vi "HelioNoise.vi"() -> ()   [LabVIEW 2010]
uses:
  bricks/classes/ImageCollection/ImageCollection.lvclass
  <vilib>/Analysis/NI_AALBase.lvlib
  bricks/classes/ImageCollection/add_mode_enum.ctl
  bricks/classes/Image/Image.lvclass
  bricks/classes/Image/storage_mode.ctl
  <vilib>/vision/Image Controls.llb/IMAQ Image.ctl
panel:
  in  "loadROIsButton":bool
  in  "saveROIsButton":bool
  out "DS/S vs. S (bg subtracted)":cluster{dbl, dbl}[](graph) caption="DS/S vs. S (background subtracted)"
  in  "saveButton":bool
  out "files to process":i32
  out "progress":u8(slide) scale=0.0..100.0
  in  "pattern":string="*channel01.tif"
  out "ROIs":T1(plugin-control)
  out "DS/S vs. S (bg NOT subtracted)":cluster{dbl, dbl}[](graph) caption="DS/S vs. S (background NOT subtracted from S)"
  in  "stopButton":bool
  in  "path":path
  in  "runButton":bool
  # "Noise Analyser"
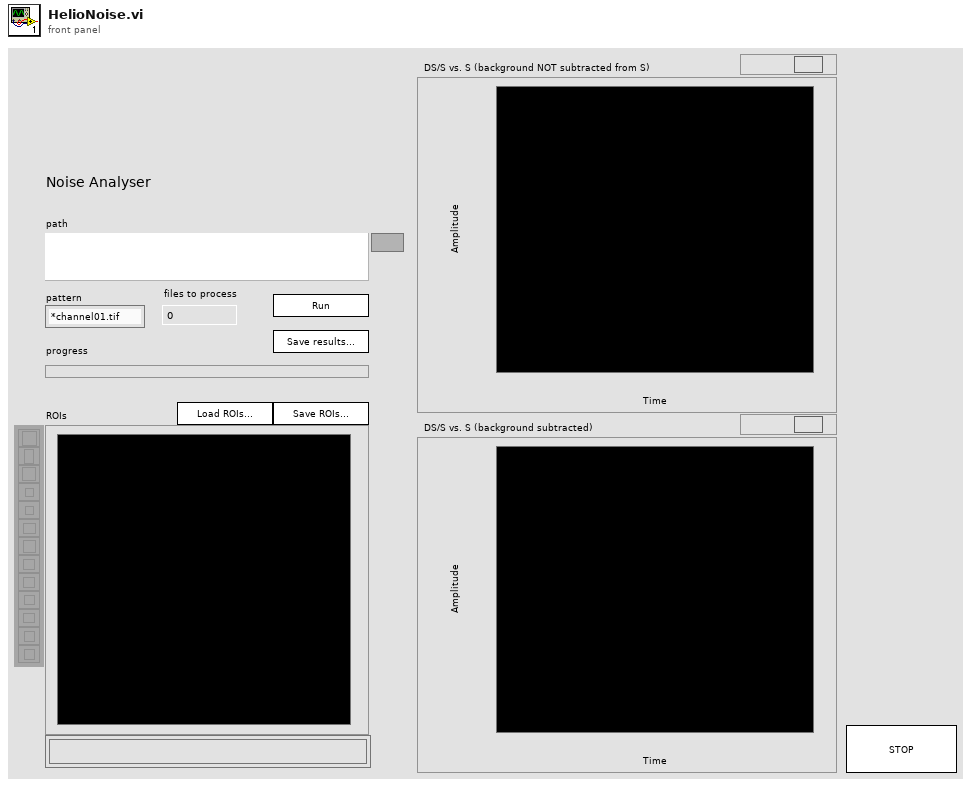
[diagram p1: front panel]
types:
  T1 = typedef "IMAQ Image.ctl" = refnum<image>
  T2 = typedef "Image.lvclass/storage_mode.ctl" = enum16{"RAM", "disk"}
  T3 = typedef "ImageCollection.lvclass/add_mode_enum.ctl" = enum16{"instance", "copy"}
  T4 = typedef "ROI Descriptor" = cluster{"Global Rectangle":i32[], "Contours":cluster{"ID":enum32{"External", "Internal"}, "Type":u32, "Coordinates":i32[]}[]}
  T5 = cluster{"Global Rectangle":i32[], "Contours":cluster{"Contour Type":u32, "ROI Type":u32, "Points":i32[]}[]}
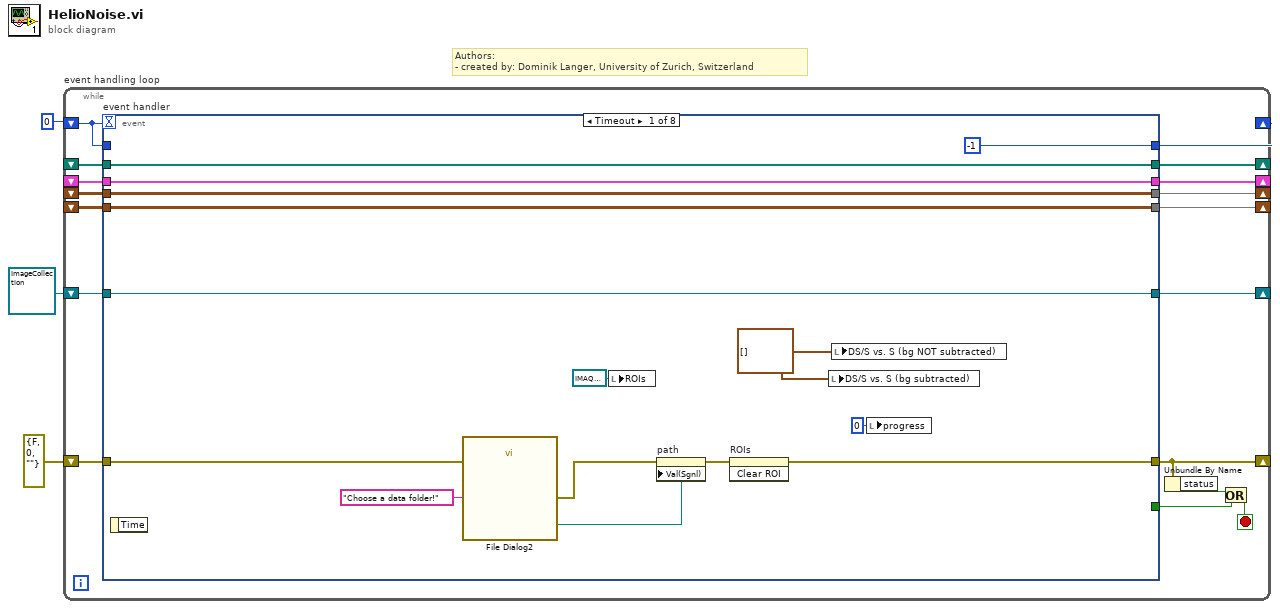
[diagram p0: block diagram]
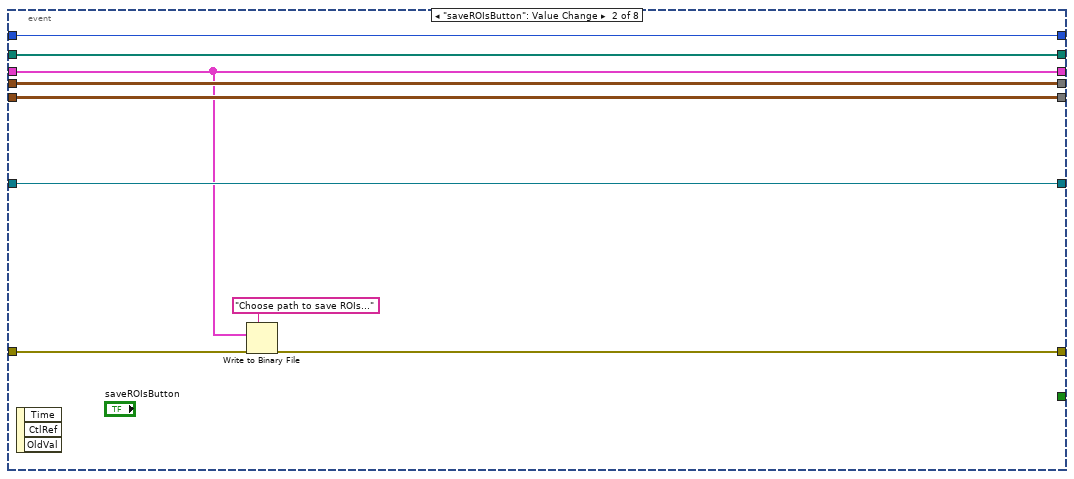
[diagram p2: hidden frame]
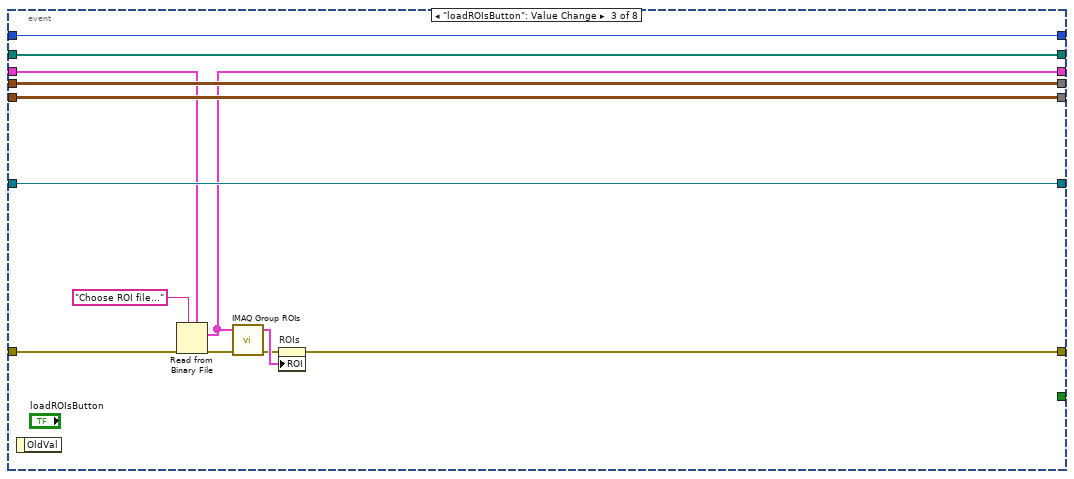
[diagram p3: hidden frame]
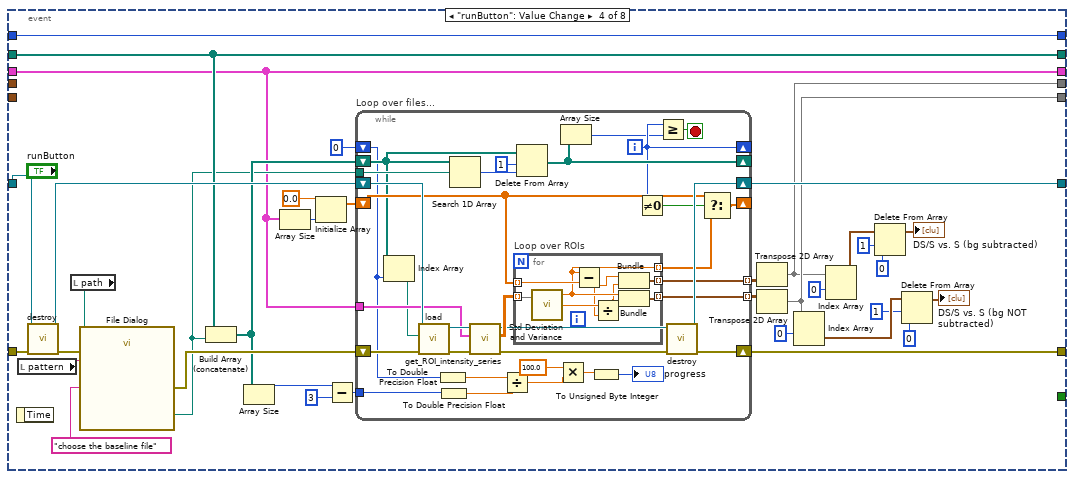
[diagram p4: hidden frame]
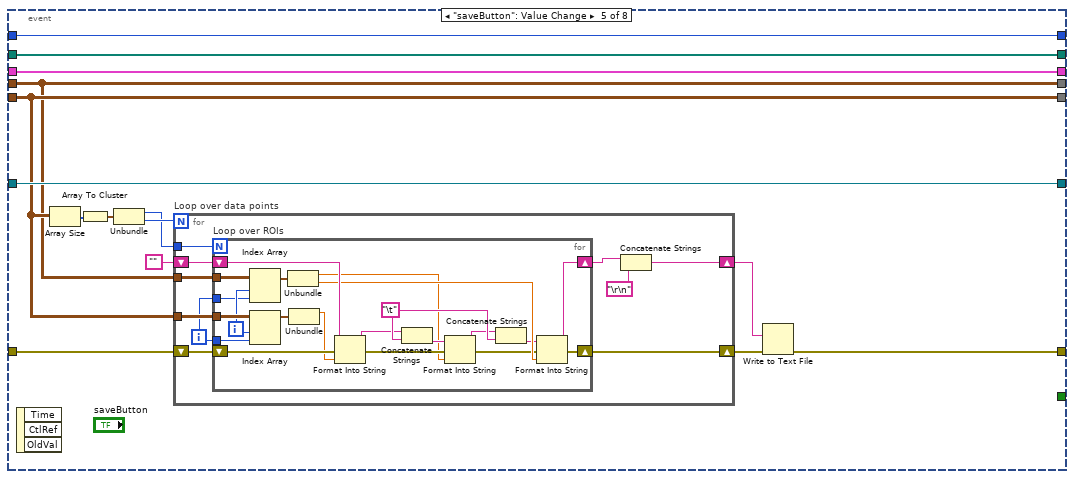
[diagram p5: hidden frame]
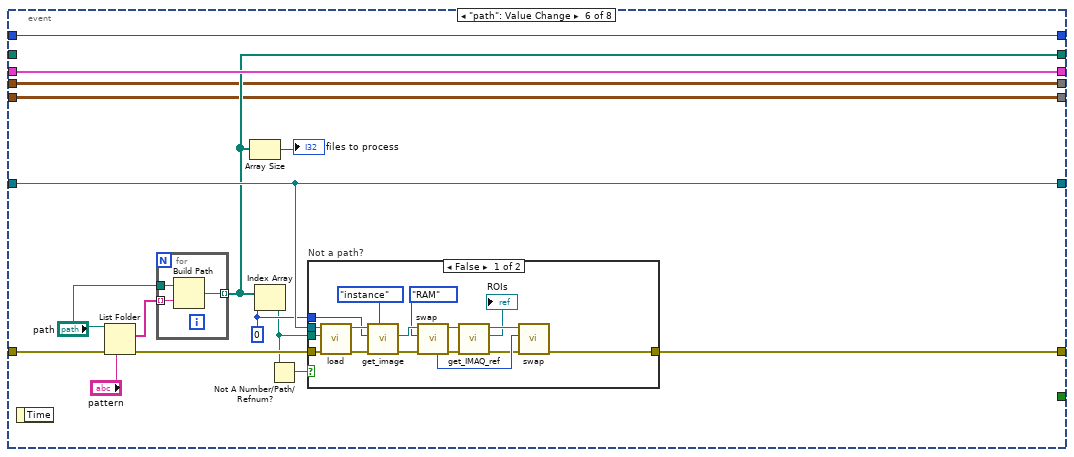
[diagram p6: hidden frame]
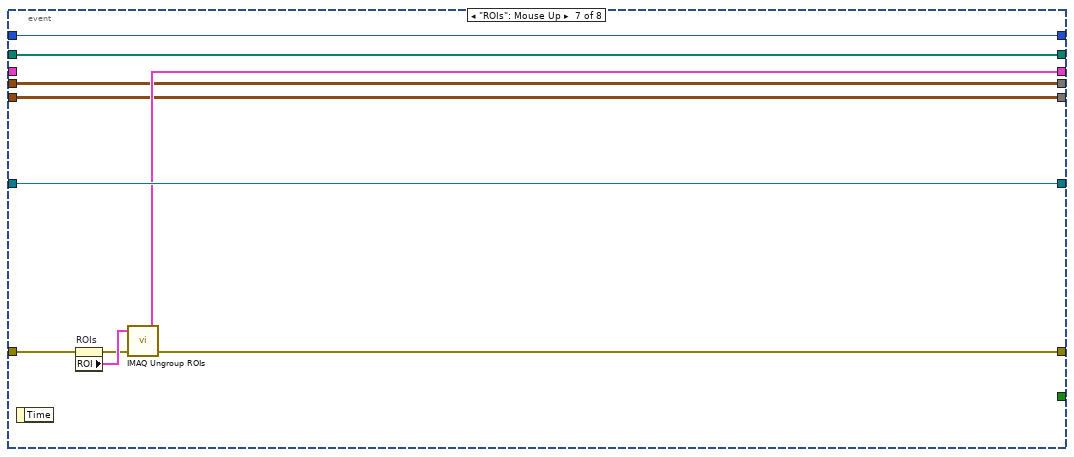
[diagram p8: hidden frame]
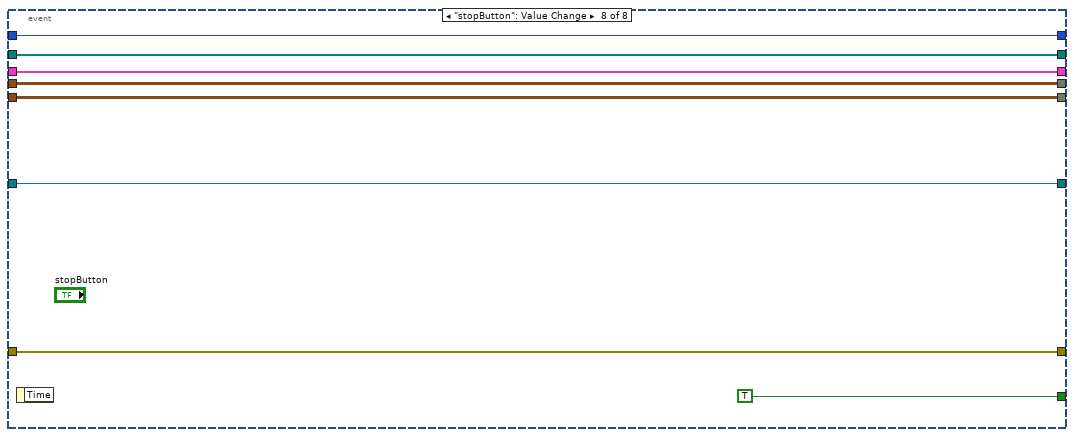
[diagram p9: hidden frame]
diagram:
  # "Authors: \n- created by: Dominik Langer, University of Zurich, Switzerland"
  n1 = while "event handling loop" {
    shift-right: [w15] -> _
    shift-left: errorcluster {"status"=FALSE, "code"=0, "source"=""} ("error out") -> [w19]
    shift-right: [w18] -> _
    shift-left: refnum<class "ImageCollection.lvclass"> refnum ("ImageCollection.lvclass") -> [w20]
    shift-right: [w16] -> _
    shift-left: _ -> [w17]
    shift-right: [w10] -> _
    shift-left: 0 -> [w11]
    shift-right: [w9] -> _
    shift-left: _ -> [w8]
    shift-right: [w6] -> _
    shift-left: _ -> [w7]
    shift-right: [w5] -> _
    shift-left: _ -> [w4]
    stop <- w12 stop-if-true
    n2 = event "event handler" shown="[0] Timeout" {
      selector: _ -> [_ _ _ _ _ _ _ _]
      dyn-events: _ -> [_ _ _ _ _ _ _ _]
      timeout: w11 -> [_ _ _ _ _ _ _ _]
      tunnel: w20 -> [w35 w44 w57 w89 w149 w192 w227 w234]
      tunnel: w19 -> [w27 w39 w52 w90 w144 w196 w226 w235]
      tunnel: [w22 w38 w49 w93 w142 w190 w223 w235] -> w15
      tunnel: [w35 w44 w57 w92 w149 w192 w227 w234] -> w18
      tunnel: [_ _ _ _ _ _ _ TRUE] -> w14
      tunnel: w17 -> [w34 w43 w56 w83 w148 _ w222 w232]
      tunnel: [w34 w43 w56 w83 w148 w184 w222 w232] -> w16
      tunnel: [-1 w42 w55 w91 w147 w186 w221 w231] -> w10
      tunnel: w11 -> [_ w42 w55 w91 w147 w186 w221 w231]
      tunnel: [w31 w37 w48 w72 w146 w185 w220 w230] -> w9
      tunnel: w8 -> [w31 w37 w51 w72 w146 w185 _ w230]
      tunnel: w7 -> [w29 w41 w54 _ w140 w182 w219 w229]
      tunnel: [w29 w41 w54 w68 w140 w182 w219 w229] -> w6
      tunnel: [w28 w40 w53 w60 w135 w181 w218 w228] -> w5
      tunnel: w4 -> [w28 w40 w53 _ w135 w181 w218 w228]
      event Timeout {
        w21 = cluster{dbl, dbl}[] [] ("XY Graph")
        n3 = event-data() -> ()  [unwired: 1 in, 1 out]
        n4 = call "File Dialog2"("prompt"="Choose a data folder!", "error in"=w27) -> ("selected path"=w25:path, "error out"=w26:errorcluster)  [unwired: 10 in, 2 out]
        n5 = local write "ROIs"(T1 refnum ("Image")) -> ()
        n6 = property on="path" class="Path"(error in=w26, "Val(Sgnl)"=w25) -> (error out=w23:errorcluster)  [unwired: 1 in, 1 out]
        n7 = invoke on="ROIs" class="ImageControl" method="Clear ROI"(error in=w23) -> (error out=w22:errorcluster)  [unwired: 2 in, 2 out]
        n8 = local write "DS/S vs. S (bg subtracted)"(w21) -> ()
        n9 = local write "DS/S vs. S (bg NOT subtracted)"(w21) -> ()
        n10 = local write "progress"(u8 0 ("progress")) -> ()
      }
      event "saveROIsButton": Value Change {
        n11 = event-data() -> ()  [unwired: 1 in, 3 out]
        n12 = Write to Binary File(data=w37, error in=w39, 7:"Choose path to save ROIs..." ("prompt (Choose or enter file path)")) -> (error out=w38:errorcluster)  [unwired: 3 in, 2 out]
      }
      event "loadROIsButton": Value Change {
        n13 = event-data() -> ()  [unwired: 1 in, 1 out]
        n14 = Read from Binary File(5:w51, 7:"Choose ROI file..." ("prompt (Open existing file)"), 8:w52) -> (0:w46:errorcluster, 2:w48:T4[])  [unwired: 3 in, 2 out]
        n15 = call "IMAQ Group ROIs"("error in (no error)"=w46, "ROI Descriptors"=w48) -> ("error out"=w45:errorcluster, "ROI Descriptor out"=w47:T4)  [unwired: 2 in]
        n16 = property on="ROIs" class="ImageControl"(error in=w45, "ROI"=w47) -> (error out=w49:errorcluster)  [unwired: 1 in, 1 out]
      }
      event "runButton": Value Change {
        n17 = event-data() -> ()  [unwired: 1 in, 1 out]
        n18 = local read "pattern"() -> (w77:string)
        n19 = call-dynamic "destroy.vi"("error in (no error)"=w90, "ImageCollection in"=w89) -> ("error out"=w85:errorcluster, "ImageCollection out"=w88:refnum<class "ImageCollection.lvclass">)  [unwired: 8 in]
        n20 = local read "path"() -> (w78:path)
        n21 = call "File Dialog"("start path"=w78, "prompt"="choose the baseline file", "error in"=w85, "pattern (all files)"=w77) -> ("selected path"=w75:path, "error out"=w84:errorcluster)  [unwired: 8 in, 2 out]
        n22 = Build Array (concatenate)(w83, w75) -> (w76:path[])
        n23 = Array Size(array=w76) -> (size(s)=w66:i32)
        n24 = Array Size(array=w72) -> (size(s)=w73:i32)
        n25 = Initialize Array(0.0 ("element"), w73) -> (w70:dbl[])
        n26 = Subtract(x=w66, y=3) -> (x-y=w65:i32)
        n27 = while "Loop over files..." {
          shift-right: [w120] -> w93
          shift-left: w84 -> [w125]
          tunnel: [w108] -> w87 mode=indexing
          shift-right: [w118] -> w92
          shift-left: w88 -> [w126]
          tunnel: w72 -> [w117]
          shift-right: [w109] -> _
          shift-left: w70 -> [w107]
          shift-right: [w99] -> _
          shift-left: w76 -> [w103]
          tunnel: w75 -> [w106]
          shift-right: [w98] -> _
          shift-left: 0 -> [w100]
          tunnel: w65 -> [w95]
          tunnel: [w94] -> w64 mode=indexing
          i -> [w98]
          stop <- w97 stop-if-true
          n28 = Index Array(array=w103, index=w100) -> (element=w102:path)
          n29 = call "load.vi"("error in (no error)"=w125, "Path"=w102, "ImageCollection in"=w126) -> ("error out"=w124:errorcluster, "ImageCollection out"=w123:refnum<class "ImageCollection.lvclass">)  [unwired: 5 in, 2 out]
          n30 = To Double Precision Float(number=w100) -> (double precision float=w116:dbl)
          n31 = To Double Precision Float(number=w95) -> (double precision float=w115:dbl)
          n32 = Search 1D Array(1D array=w103, element=w106) -> (index of element=w105:i32)  [unwired: 1 in]
          n33 = call "get_ROI_intensity_series.vi"("error in (no error)"=w124, "ROIs"=w117, "ImageCollection in"=w123) -> ("error out"=w121:errorcluster, "intensity series"=w122:dbl[][], "ImageCollection out"=w119:refnum<class "ImageCollection.lvclass">)  [unwired: 6 in]
          n34 = Divide(x=w116, y=w115) -> (x/y=w114:dbl)
          n35 = for "Loop over ROIs" {
            tunnel: w122 -> [w134] mode=indexing
            tunnel: [w131] -> w108 mode=indexing
            tunnel: [w130] -> w110 mode=indexing
            tunnel: w107 -> [w133] mode=indexing
            tunnel: [w129] -> w94 mode=indexing
            n36 = call <vilib>:"Std Deviation and Variance.vi"("X"=w134) -> ("mean"=w130:dbl, "standard deviation"=w132:dbl)  [unwired: 1 in, 1 out]
            n37 = Subtract(x=w130, y=w133) -> (x-y=w127:dbl)
            n38 = Divide(x=w132, y=w127) -> (x/y=w128:dbl)
            n39 = Bundle(w127, w128) -> (w129:cluster{dbl, dbl})  [unwired: 1 in]
            n40 = Bundle("mean"=w130, w128) -> (w131:cluster{"mean":dbl, dbl})  [unwired: 1 in]
          }
          n41 = Delete From Array(array=w103, length=1, index=w105) -> (array with subset deleted=w99:path[])  [unwired: 1 out]
          n42 = Multiply(x=100.0, y=w114) -> (x*y=w112:dbl)
          n43 = Array Size(array=w99) -> (size(s)=w96:i32)
          n44 = To Unsigned Byte Integer(number=w112) -> (unsigned 8bit integer=→"progress":u8)
          n45 = Not Equal To 0?(x=w98) -> (x != 0?=w101:bool)
          n46 = Greater Or Equal?(x=w98, y=w96) -> (x >= y?=w97:bool)
          n47 = call-dynamic "destroy.vi"("error in (no error)"=w121, "ImageCollection in"=w119) -> ("error out"=w120:errorcluster, "ImageCollection out"=w118:refnum<class "ImageCollection.lvclass">)  [unwired: 8 in]
          n48 = Select(t=w107, s=w101, f=w110) -> (s? t:f=w109:dbl[])
        }
        n49 = Transpose 2D Array(2D array=w64) -> (transposed array=w60:cluster{dbl, dbl}[][])
        n50 = Transpose 2D Array(2D array=w87) -> (transposed array=w68:cluster{"mean":dbl, dbl}[][])
        n51 = Index Array(array=w68, index (row)=0) -> (element=w82:cluster{"mean":dbl, dbl}[])  [unwired: 1 in]
        n52 = Index Array(array=w60, index (row)=0) -> (element=w58:cluster{dbl, dbl}[])  [unwired: 1 in]
        n53 = Delete From Array(array=w58, length=1, index=0) -> (array with subset deleted=→"DS/S vs. S (bg subtracted)":cluster{dbl, dbl}[])  [unwired: 1 out]
        n54 = Delete From Array(array=w82, length=1, index=0) -> (array with subset deleted=→"DS/S vs. S (bg NOT subtracted)":cluster{"mean":dbl, dbl}[])  [unwired: 1 out]
      }
      event "saveButton": Value Change {
        n55 = event-data() -> ()  [unwired: 1 in, 3 out]
        n56 = Array Size(array=w140) -> (size(s)=w139:i32[])
        n57 = Array To Cluster(array=w139) -> (cluster=w138:cluster{"[0]":i32, "[1]":i32})
        n58 = Unbundle(w138) -> ("[0]"=w136:i32, "[1]"=w137:i32)
        n59 = for "Loop over data points" {
          N: w137 -> [_]
          tunnel: w140 -> [w159]
          shift-right: [w153] -> w141
          shift-left: "" -> [w158]
          shift-right: [w156] -> w143
          shift-left: w144 -> [w157]
          tunnel: w136 -> [w155]
          tunnel: w135 -> [w151]
          i -> [w150]
          n60 = for "Loop over ROIs" {
            N: w155 -> [_]
            tunnel: w159 -> [w175]
            shift-right: [w176] -> w154
            shift-left: w158 -> [w177]
            shift-right: [w178] -> w156
            shift-left: w157 -> [w180]
            tunnel: w150 -> [w173]
            tunnel: w151 -> [w171]
            tunnel: w150 -> [w170]
            i -> [w172]
            w164 = "\t"
            n61 = Index Array(array=w171, index (row)=w172, index (col)=w170) -> (element=w169:cluster{dbl, dbl})
            n62 = Index Array(array=w175, index (row)=w172, index (col)=w173) -> (element=w174:cluster{"mean":dbl, dbl})
            n63 = Unbundle(w169) -> (w160:dbl, w168:dbl)
            n64 = Unbundle(w174) -> ("mean"=w179:dbl)  [unwired: 1 out]
            n65 = Format Into String(initial string=w177, error in=w180, w179) -> (resulting string=w162:string, error out=w167:errorcluster)  [unwired: 1 in]
            n66 = Concatenate Strings(w162, w164) -> (w165:string)
            n67 = Format Into String(initial string=w165, error in=w167, w160) -> (resulting string=w163:string, error out=w166:errorcluster)  [unwired: 1 in]
            n68 = Concatenate Strings(w163, w164) -> (w161:string)
            n69 = Format Into String(initial string=w161, error in=w166, w168) -> (resulting string=w176:string, error out=w178:errorcluster)  [unwired: 1 in]
          }
          n70 = Concatenate Strings(w154, "\r\n") -> (w153:string)
        }
        n71 = Write to Text File(text=w141, error in=w143) -> (error out=w142:errorcluster)  [unwired: 2 in, 2 out]
      }
      event "path": Value Change {
        w191 = 0 ("index")
        n72 = event-data() -> ()  [unwired: 1 in, 1 out]
        n73 = List Folder(path="path", pattern="pattern", error in=w196) -> (filenames=w195:string[], error out=w193:errorcluster)  [unwired: 1 in, 2 out]
        n74 = for {
          tunnel: w195 -> [w217] mode=indexing
          tunnel: "path" -> [w216]
          tunnel: [w215] -> w184 mode=indexing
          n75 = Build Path(base path=w216, name or relative path=w217) -> (appended path=w215:path)
        }
        n76 = Array Size(array=w184) -> (size(s)=→"files to process":i32)
        n77 = Index Array(array=w184, index=w191) -> (element=w188:path)
        n78 = Not A Number/Path/Refnum?(number/path/refnum=w188) -> (NaN/Path/Refnum?=w187:bool)
        n79 = case "Not a path?" shown="False" w187 {
          tunnel: w193 -> [w213 w214]
          tunnel: w192 -> [w212 _]
          tunnel: w191 -> [w209 _]
          tunnel: [w199 w214] -> w190
          tunnel: w188 -> [w200 _]
          frame False {
            n80 = call "load.vi"("error in (no error)"=w213, "Path"=w200, "ImageCollection in"=w212) -> ("error out"=w211:errorcluster, "ImageCollection out"=w210:refnum<class "ImageCollection.lvclass">)  [unwired: 5 in, 2 out]
            n81 = call-dynamic "get_image.vi"("get image as..."=add_mode_enum."instance", "error in (no error)"=w211, "index"=w209, "ImageCollection in"=w210) -> ("error out"=w207:errorcluster, "Image.lvclass"=w205:refnum<class "Image.lvclass">)  [unwired: 5 in, 1 out]
            n82 = call-dynamic "swap.vi"("error in (no error)"=w207, "storage type target"=storage_mode."RAM", "Image in"=w205) -> ("error out"=w206:errorcluster, "Image out"=w204:refnum<class "Image.lvclass">, "previous storage mode"=w202:T2)  [unwired: 6 in]
            n83 = call-dynamic "get_IMAQ_ref.vi"("error in (no error)"=w206, "Image.lvclass in"=w204) -> ("error out"=w197:errorcluster, "Image"=→"ROIs":T1, "Image.lvclass out"=w203:refnum<class "Image.lvclass">)  [unwired: 6 in, 1 out]
            n84 = call-dynamic "swap.vi"("error in (no error)"=w197, "storage type target"=w202, "Image in"=w203) -> ("error out"=w199:errorcluster)  [unwired: 6 in, 2 out]
          }
          frame True {
          }
        }
      }
      event "ROIs": Mouse Up {
        n85 = event-data() -> ()  [unwired: 1 in, 1 out]
        n86 = property on="ROIs" class="ImageControl"(error in=w226) -> (error out=w224:errorcluster, "ROI"=w225:T5)  [unwired: 1 in, 1 out]
        n87 = call "IMAQ Ungroup ROIs"("error in (no error)"=w224, "ROI Descriptor"=w225) -> ("error out"=w223:errorcluster, "ROI Descriptors out"=w220:T4[])  [unwired: 2 in]
      }
      event "stopButton": Value Change {
        n88 = event-data() -> ()  [unwired: 1 in, 1 out]
      }
    }
    n89 = Unbundle By Name(w15) -> ("status"=w13:bool)
    n90 = Or(x=w13, y=w14) -> (x .or. y?=w12:bool)
  }
